vi "Generate Waveform.vi"(8 "error in (no error)":errorcluster, 10 "Voice Level Controls in":variant, 11 "MIDI Controls in":variant) -> (0 "error out":errorcluster, 2 "Signal Generation out":variant)   [LabVIEW 2014, in "mySynthesizer.lvlib" / "Signal Generation.lvlib"]
uses:
  Signal Generation/Signal Generation.lvlib
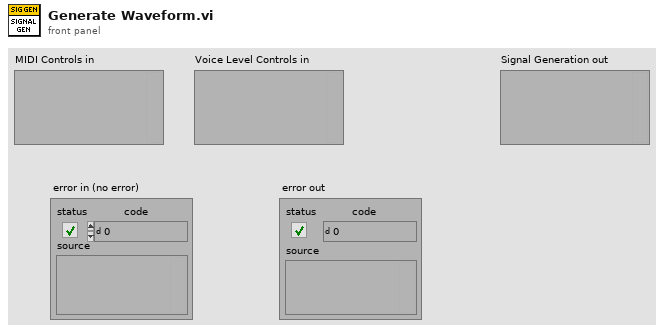
[diagram p1: front panel]
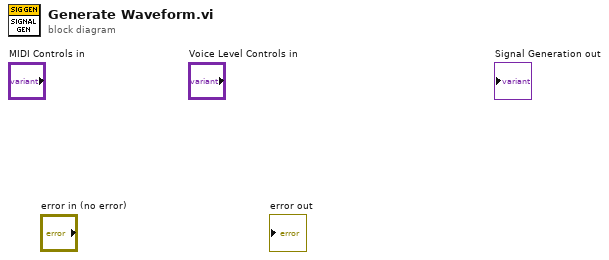
[diagram p0: block diagram]
diagram:
